vi "Save Object.vi"(8 "error in (no error)":errorcluster, 10 "Object":T1={"Name"="", "Is Acquired"=FALSE, "Queue"=refnum, "Message To Send"={"Enqueuer"=refnum, "Message"=refnum}, "Save Parameters"=variant(bool FALSE)}, 11 "StorageService in":refnum<class "StorageService.lvclass">) -> (0 "error out":errorcluster, 3 "StorageService out":refnum<class "StorageService.lvclass">)   [LabVIEW 2014, in "StorageService.lvclass"]
uses:
  StorageService.lvclass
  RegisteredObject.ctl
  <vilib>/ActorFramework/Message Enqueuer/Message Enqueuer.lvclass
  Model/ReplayData Msg/ReplayData Msg.lvclass
  Model/Data/AbstractData/AbstractData.lvclass
  StorageService.lvclass/StorageService.ctl
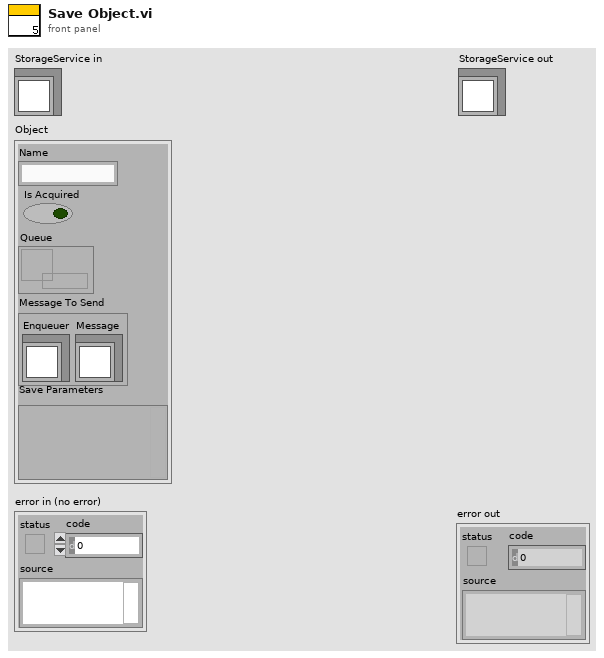
[diagram p1: front panel]
types:
  T1 = typedef "StorageService.lvclass/RegisteredObject.ctl" = cluster{"Name":string, "Is Acquired":bool, "Queue":refnum<queue>, "Message To Send":cluster{"Enqueuer":refnum<class "Message Enqueuer.lvclass">, "Message":refnum<class "ReplayData Msg.lvclass">}, "Save Parameters":variant}
  T2 = enum16{"open", "replace", "create", "open or create", "replace or create", "replace or create with confirmation"}
  T3 = cluster{"Data":refnum<class "AbstractData.lvclass">, "Parameter":refnum<class "AbstractData.lvclass">}[]
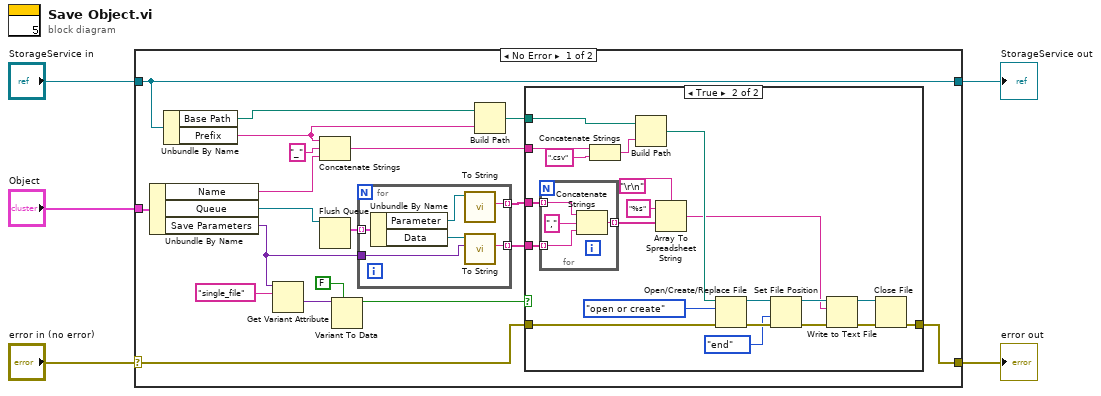
[diagram p0: block diagram]
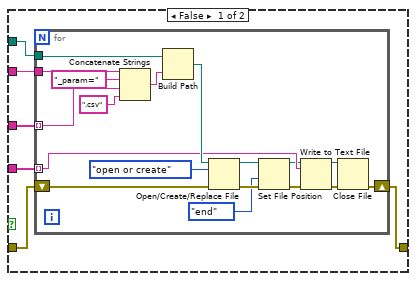
[diagram p2: hidden frame]
diagram:
  n1 = case shown="No Error" "error in (no error)" {
    selector: "error in (no error)" -> [w17 w81]
    tunnel: [w15 w81] -> w4
    tunnel: [w16 w80] -> w2
    tunnel: "StorageService in" -> [w16 w80]
    tunnel: "Object" -> [w24 _]
    frame No Error {
      n2 = Unbundle By Name(w24) -> ("Name"=w14:string, "Queue"=w22:refnum<queue>, "Save Parameters"=w9:variant)
      n3 = Unbundle By Name(w16) -> ("Base Path"=w8:path, "Prefix"=w6:string)
      n4 = Get Variant Attribute(Variant=w9, name="single_file") -> (value=w12:variant)  [unwired: 2 in, 3 out]
      n5 = Concatenate Strings(w6, "_" ("string"), w14) -> (w21:string)
      n6 = Flush Queue(queue=w22) -> (remaining elements=w20:T3)  [unwired: 1 in, 2 out]
      n7 = Variant To Data(type=FALSE, Variant=w12) -> (data=w11:bool)  [unwired: 1 in, 1 out]
      n8 = for {
        tunnel: [w28] -> w18 mode=indexing
        tunnel: [w27] -> w19 mode=indexing
        tunnel: w20 -> [w26] mode=indexing
        tunnel: w9 -> [w25]
        n9 = Unbundle By Name(w26) -> ("Parameter"=w30:refnum<class "AbstractData.lvclass">, "Data"=w29:refnum<class "AbstractData.lvclass">)
        n10 = call-dynamic "To String.vi"("AbstractData in"=w30) -> ("String"=w28:string)  [unwired: 8 in, 2 out]
        n11 = call-dynamic "To String.vi"("Parameters"=w25, "AbstractData in"=w29) -> ("String"=w27:string)  [unwired: 7 in, 2 out]
      }
      n12 = Build Path(base path=w8, name or relative path=w6) -> (appended path=w7:path)
      n13 = case shown="True" w11 {
        tunnel: w21 -> [w33 w74]
        tunnel: w7 -> [w34 w75]
        tunnel: w19 -> [w35 w70]
        tunnel: w18 -> [w36 w71]
        tunnel: w17 -> [w32 w64]
        tunnel: [w31 w63] -> w15
        frame False {
          n14 = for {
            tunnel: w36 -> [w50] mode=indexing
            tunnel: w35 -> [w43] mode=indexing
            tunnel: w34 -> [w53]
            tunnel: w33 -> [w52]
            shift-right: [w46] -> w31
            shift-left: w32 -> [w45]
            n15 = Concatenate Strings(w52, "_param=" ("string"), w50, ".csv" ("string")) -> (w54:string)
            n16 = Build Path(base path=w53, name or relative path=w54) -> (appended path=w44:path)
            n17 = Open/Create/Replace File(file path (use dialog)=w44, error in=w45, operation (0:open)=T2."open or create") -> (refnum out=w41:refnum<file>, error out=w39:errorcluster)  [unwired: 3 in, 1 out]
            n18 = Set File Position(refnum=w41, from (0:start)=enum16{"start", "end", "current"}."end", error in=w39) -> (refnum out=w40:refnum<file>, error out=w38:errorcluster)  [unwired: 1 in]
            n19 = Write to Text File(file (use dialog)=w40, text=w43, error in=w38) -> (refnum out=w47:refnum<file>, error out=w48:errorcluster)  [unwired: 1 in, 1 out]
            n20 = Close File(refnum=w47, error in=w48) -> (error out=w46:errorcluster)  [unwired: 1 out]
          }
        }
        frame True {
          n21 = for {
            tunnel: w71 -> [w79] mode=indexing
            tunnel: w70 -> [w78] mode=indexing
            tunnel: [w77] -> w69 mode=indexing
            n22 = Concatenate Strings(w79, ",", w78) -> (w77:string)
          }
          n23 = Concatenate Strings(w74, ".csv" ("string")) -> (w73:string)
          n24 = Build Path(base path=w75, name or relative path=w73) -> (appended path=w67:path)
          n25 = Array To Spreadsheet String(delimiter (Tab)="\r\n", array=w69, 3:"%s" ("format string")) -> (spreadsheet string=w55:string)
          n26 = Open/Create/Replace File(file path (use dialog)=w67, error in=w64, operation (0:open)=T2."open or create") -> (refnum out=w58:refnum<file>, error out=w60:errorcluster)  [unwired: 3 in, 1 out]
          n27 = Set File Position(refnum=w58, from (0:start)=enum16{"start", "end", "current"}."end", error in=w60) -> (refnum out=w57:refnum<file>, error out=w59:errorcluster)  [unwired: 1 in]
          n28 = Write to Text File(file (use dialog)=w57, text=w55, error in=w59) -> (refnum out=w66:refnum<file>, error out=w65:errorcluster)  [unwired: 1 in, 1 out]
          n29 = Close File(refnum=w66, error in=w65) -> (error out=w63:errorcluster)  [unwired: 1 out]
        }
      }
    }
    frame Error {
    }
  }
  "error out" <- w4
  "StorageService out" <- w2
